vi "Add New Message.vi"(8 "error in (no error)":errorcluster, 11 "Node Ptr":u64 format="%.0x") -> (0 "error out":errorcluster)   [LabVIEW 2020, in "Instrument Addon System Explorer.lvlib"]
uses:
  Instrument Addon System Explorer.lvlib
  APIs/Scripting API/TypeDefs/Message Settings.ctl
  APIs/Scripting API/TypeDefs/Protection Types.ctl
  Addon Shared/SubVIs/Constants.vi
  APIs/Scripting API/Messages/Create Message - Trigger Only.vi
  Addon Shared/Instrument Addon Shared.lvlib
  APIs/Scripting API/Instrument Addon Scripting API.lvlib
  <vilib>/NI VeriStand/Custom Device API/Custom Device API.lvlib
panel:
  in  "Tag":string
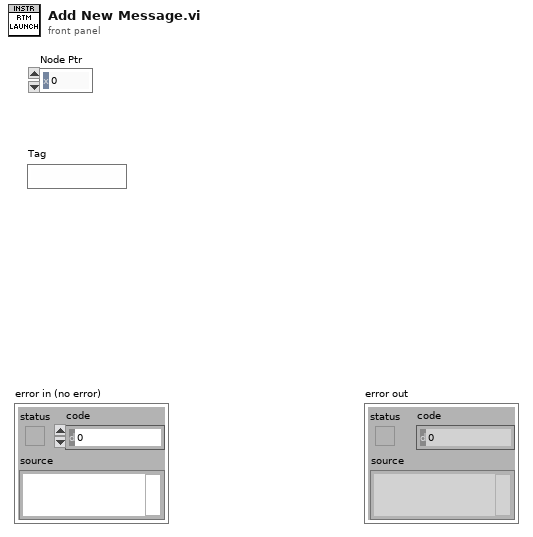
[diagram p1: front panel]
types:
  T1 = typedef "Instrument Addon Scripting API.lvlib/Message Settings.ctl" = cluster{"Protection":T2, "Enable Periodic Default":bool, "Trigger Channel refnum":u64}
  T2 = typedef "Instrument Addon Scripting API.lvlib/Protection Types.ctl" = enum16{"None", "CRC-32", "Checksum U16", "Checksum U32", "Checksum U8"}
  T3 = typedef "Custom Device API.lvlib/Custom Device Item Ref.ctl" = u64
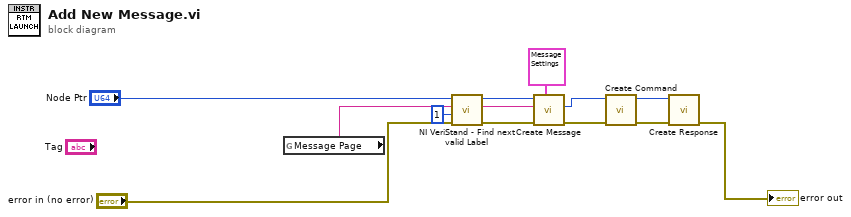
[diagram p0: block diagram]
diagram:
  n1 = global read "Constants.vi" "Message Page"() -> (w4:string)
  n2 = call <vilib>:"NI VeriStand - Find next valid Label.vi"("error in (no error)"="error in (no error)", "Start Value (1)"=1, "Label"=w4, "Item Ref in"="Node Ptr") -> ("error out"=w2:errorcluster, "Label out"=w1:string, "Item Ref out"=w3:T3)  [unwired: 3 in, 2 out]
  n3 = call-poly "Create Message.vi"("optional settings"=T1 {"Protection"=enum."None", "Enable Periodic Default"=FALSE, "Trigger Channel refnum"=18446744073709551615} ("Message Settings"), "error in (no error)"=w2, "message name"=w1, "message group refnum in"=w3) -> ("error out"=w12:errorcluster, "message refnum out"=w11:T3)  [unwired: 5 in, 1 out]
  n4 = call "Create Command.vi"("error in"=w12, "message refnum In"=w11) -> ("error out"=w10:errorcluster, "message refnum out"=w9:T3)  [unwired: 7 in, 1 out]
  n5 = call "Create Response.vi"("error in (no error)"=w10, "message refnum in"=w9) -> ("error out"=→"error out":errorcluster)  [unwired: 7 in, 2 out]
